vi "Translate 1D indexes to 2D.vi"(8 "error in (no error)":errorcluster, 10 "Range Array for Queue size mapping":refnum<class "2D Array s64.lvclass">, 11 "1D Indexes in":refnum<class "1D Array u32.lvclass">) -> (0 "error out":errorcluster, 3 "Mapped to 2D indexes out":refnum<class "1D Array s32.lvclass">)   [LabVIEW 2020, in "G2CPU Line Profile.lvlib"]
uses:
  G2CPU Line Profile.lvlib
  <vilib>/Natan Biesmans/G2CPU GPU and CPU HPC Toolkit/G2CPU Libraries/Arrays/1DArray/u32/1D Array u32.lvclass
  C:/Program Files/National Instruments/LabVIEW 2025/vi.lib/Natan Biesmans/G2CPU GPU and CPU HPC Toolkit/G2CPU Libraries/Arrays/Array/Array Prototype.lvclass
  <vilib>/Natan Biesmans/G2CPU GPU and CPU HPC Toolkit/G2CPU Libraries/Arrays/2DArray/s64/2D Array s64.lvclass
  <vilib>/Natan Biesmans/G2CPU GPU and CPU HPC Toolkit/G2CPU Libraries/Arrays/1DArray/s32/1D Array s32.lvclass
  <vilib>/Natan Biesmans/G2CPU GPU and CPU HPC Toolkit/G2CPU Libraries/Arrays/Array/Array Prototype.lvclass/Array Prototype.ctl
  3cda7c46-1737-42c5-90ff-c6c13540a65e.vi
  28bd746a-8bdf-434a-83c2-b49bf21645d8.vi
  78b6c921-1702-49f5-a8de-ca7d67101d2e.vi
  74281535-8ec9-475a-9c6f-61cdcc5771e7.vi
  da6a37ee-0c13-4542-a02e-82ed8c504917.vi
  f0154963-fb83-49e6-af23-53d56b8f6f43.vi
  fa8fd128-a982-493c-bb6b-fb6c2fa3ced3.vi
  dd97a9ad-5d19-4764-bb21-7805c3de5fd8.vi
  <vilib>/Natan Biesmans/G2CPU GPU and CPU HPC Toolkit/G2CPU Libraries/Arrays/Array/G2CPU Get Array Pointer.vi
  3cda7c46-1737-42c5-90ff-c6c13540a65e.vi/e7247370-a01f-465a-ac0e-4dfefcb1bb87.vi
  3cda7c46-1737-42c5-90ff-c6c13540a65e.vi/345e91f0-9a5e-4de4-af9c-133346717e4a.vi
  28bd746a-8bdf-434a-83c2-b49bf21645d8.vi/e7247370-a01f-465a-ac0e-4dfefcb1bb87.vi
  28bd746a-8bdf-434a-83c2-b49bf21645d8.vi/345e91f0-9a5e-4de4-af9c-133346717e4a.vi
  78b6c921-1702-49f5-a8de-ca7d67101d2e.vi/008596a2-72c7-4b94-8d63-a430db0cac39.vi
  78b6c921-1702-49f5-a8de-ca7d67101d2e.vi/d781c0aa-35dc-4978-ac14-8fc3832ba4f0.vi
  78b6c921-1702-49f5-a8de-ca7d67101d2e.vi/5ea8fe8e-4ffc-4d1c-84a0-6eba72fe9718.vi
  78b6c921-1702-49f5-a8de-ca7d67101d2e.vi/e2c9d363-485e-46f6-8192-2d8aa165dabd.vi
  78b6c921-1702-49f5-a8de-ca7d67101d2e.vi/677e326b-dc8f-4d68-b1d9-971c0162f72d.vi
  74281535-8ec9-475a-9c6f-61cdcc5771e7.vi/e2c9d363-485e-46f6-8192-2d8aa165dabd.vi
  74281535-8ec9-475a-9c6f-61cdcc5771e7.vi/677e326b-dc8f-4d68-b1d9-971c0162f72d.vi
  da6a37ee-0c13-4542-a02e-82ed8c504917.vi/5793b77b-c002-4ebf-9075-685617c95341.vi
  da6a37ee-0c13-4542-a02e-82ed8c504917.vi/2ed3ef86-c00d-4d71-b84c-20267a6dfcf9.vi
  f0154963-fb83-49e6-af23-53d56b8f6f43.vi/cfed8f62-9c64-4dab-912e-5e7c21cb720b.vi
  fa8fd128-a982-493c-bb6b-fb6c2fa3ced3.vi/5793b77b-c002-4ebf-9075-685617c95341.vi
  fa8fd128-a982-493c-bb6b-fb6c2fa3ced3.vi/2ed3ef86-c00d-4d71-b84c-20267a6dfcf9.vi
  dd97a9ad-5d19-4764-bb21-7805c3de5fd8.vi/9d769ba4-bbb4-4eb6-9175-95d7d139327c.vi
  dd97a9ad-5d19-4764-bb21-7805c3de5fd8.vi/8bfea9e7-a130-4d69-b32e-15c58d17157f.vi
  dd97a9ad-5d19-4764-bb21-7805c3de5fd8.vi/25f1b8bb-c437-45f4-b6eb-f3e32cc20aa5.vi
  dd97a9ad-5d19-4764-bb21-7805c3de5fd8.vi/309f54b5-9a40-4a1d-900d-2d620fefb202.vi
  da6a37ee-0c13-4542-a02e-82ed8c504917.vi/5793b77b-c002-4ebf-9075-685617c95341.vi/3e802c67-fb96-46a3-ae13-4994a8508b4f.vi
  da6a37ee-0c13-4542-a02e-82ed8c504917.vi/5793b77b-c002-4ebf-9075-685617c95341.vi/5a50fc67-79e7-4972-80c2-92243cd53dd4.vi
  da6a37ee-0c13-4542-a02e-82ed8c504917.vi/5793b77b-c002-4ebf-9075-685617c95341.vi/4b7910ad-0c4a-46e4-b1b3-c9721aeaa91e.vi
  da6a37ee-0c13-4542-a02e-82ed8c504917.vi/2ed3ef86-c00d-4d71-b84c-20267a6dfcf9.vi/730f6c57-5c0b-4ee9-b61e-75067b25222b.vi
  da6a37ee-0c13-4542-a02e-82ed8c504917.vi/2ed3ef86-c00d-4d71-b84c-20267a6dfcf9.vi/096b8799-7810-404e-baca-ba9279cec4bd.vi
  da6a37ee-0c13-4542-a02e-82ed8c504917.vi/2ed3ef86-c00d-4d71-b84c-20267a6dfcf9.vi/0f1a5a47-bcc5-4796-ac31-8dfcfbc0d7d1.vi
  da6a37ee-0c13-4542-a02e-82ed8c504917.vi/2ed3ef86-c00d-4d71-b84c-20267a6dfcf9.vi/89f12e17-3330-4b72-ad8f-8dd636660732.vi
  f0154963-fb83-49e6-af23-53d56b8f6f43.vi/cfed8f62-9c64-4dab-912e-5e7c21cb720b.vi/77c7badc-ed81-4514-99c1-20d37f4e5ecc.vi
  f0154963-fb83-49e6-af23-53d56b8f6f43.vi/cfed8f62-9c64-4dab-912e-5e7c21cb720b.vi/eb76fa01-6782-47b4-b34f-9eb474c9cc78.vi
  <vilib>/Natan Biesmans/G2CPU GPU and CPU HPC Toolkit/ArrayFire Driver/VIs/Run as Multi Device.vi
  fa8fd128-a982-493c-bb6b-fb6c2fa3ced3.vi/5793b77b-c002-4ebf-9075-685617c95341.vi/3e802c67-fb96-46a3-ae13-4994a8508b4f.vi
  fa8fd128-a982-493c-bb6b-fb6c2fa3ced3.vi/5793b77b-c002-4ebf-9075-685617c95341.vi/5a50fc67-79e7-4972-80c2-92243cd53dd4.vi
  fa8fd128-a982-493c-bb6b-fb6c2fa3ced3.vi/2ed3ef86-c00d-4d71-b84c-20267a6dfcf9.vi/730f6c57-5c0b-4ee9-b61e-75067b25222b.vi
  fa8fd128-a982-493c-bb6b-fb6c2fa3ced3.vi/2ed3ef86-c00d-4d71-b84c-20267a6dfcf9.vi/096b8799-7810-404e-baca-ba9279cec4bd.vi
  fa8fd128-a982-493c-bb6b-fb6c2fa3ced3.vi/2ed3ef86-c00d-4d71-b84c-20267a6dfcf9.vi/0f1a5a47-bcc5-4796-ac31-8dfcfbc0d7d1.vi
  fa8fd128-a982-493c-bb6b-fb6c2fa3ced3.vi/2ed3ef86-c00d-4d71-b84c-20267a6dfcf9.vi/89f12e17-3330-4b72-ad8f-8dd636660732.vi
  dd97a9ad-5d19-4764-bb21-7805c3de5fd8.vi/8bfea9e7-a130-4d69-b32e-15c58d17157f.vi/edd31282-7992-4bba-af75-482693dee5e1.vi
  dd97a9ad-5d19-4764-bb21-7805c3de5fd8.vi/309f54b5-9a40-4a1d-900d-2d620fefb202.vi/730f6c57-5c0b-4ee9-b61e-75067b25222b.vi
  dd97a9ad-5d19-4764-bb21-7805c3de5fd8.vi/309f54b5-9a40-4a1d-900d-2d620fefb202.vi/096b8799-7810-404e-baca-ba9279cec4bd.vi
  dd97a9ad-5d19-4764-bb21-7805c3de5fd8.vi/309f54b5-9a40-4a1d-900d-2d620fefb202.vi/0f1a5a47-bcc5-4796-ac31-8dfcfbc0d7d1.vi
  dd97a9ad-5d19-4764-bb21-7805c3de5fd8.vi/309f54b5-9a40-4a1d-900d-2d620fefb202.vi/89f12e17-3330-4b72-ad8f-8dd636660732.vi
  da6a37ee-0c13-4542-a02e-82ed8c504917.vi/5793b77b-c002-4ebf-9075-685617c95341.vi/5a50fc67-79e7-4972-80c2-92243cd53dd4.vi/1b7cf390-2ae0-48f3-9bce-03c57eed6ee8.vi
  <vilib>/Natan Biesmans/G2CPU GPU and CPU HPC Toolkit/G2CPU Libraries/Arrays/2DArray/s32/2D Array s32.lvclass
  <vilib>/Natan Biesmans/G2CPU GPU and CPU HPC Toolkit/ArrayFire Driver/VIs/cast.vi
  <vilib>/Natan Biesmans/G2CPU GPU and CPU HPC Toolkit/G2CPU Libraries/Arrays/Array/G2CPU Set Array Pointer.vi
  <vilib>/Natan Biesmans/G2CPU GPU and CPU HPC Toolkit/ArrayFire Driver/VIs/imax.vi
  <vilib>/Natan Biesmans/G2CPU GPU and CPU HPC Toolkit/G2CPU Libraries/Arrays/SubVI/RemoveReducedDimensionForReorder.vi
  <vilib>/Natan Biesmans/G2CPU GPU and CPU HPC Toolkit/ArrayFire Driver/VIs/reorder.vi
  <vilib>/Natan Biesmans/G2CPU GPU and CPU HPC Toolkit/ArrayFire Driver/VIs/release array.vi
  <vilib>/Natan Biesmans/G2CPU GPU and CPU HPC Toolkit/ArrayFire Driver/subvi/Error Converter (ErrCode or Status).vi
  <vilib>/Natan Biesmans/G2CPU GPU and CPU HPC Toolkit/G2CPU Libraries/Arrays/SubVI/is 1D.vi
  <vilib>/Natan Biesmans/G2CPU GPU and CPU HPC Toolkit/ArrayFire Driver/VIs/add.vi
  <vilib>/Natan Biesmans/G2CPU GPU and CPU HPC Toolkit/ArrayFire Driver/VIs/iszero.vi
  <vilib>/Natan Biesmans/G2CPU GPU and CPU HPC Toolkit/ArrayFire Driver/VIs/sub.vi
  <vilib>/Natan Biesmans/G2CPU GPU and CPU HPC Toolkit/ArrayFire Driver/VIs/mod.vi
  <vilib>/Natan Biesmans/G2CPU GPU and CPU HPC Toolkit/G2CPU Libraries/Arrays/Array/Array Prototype.lvclass
  <vilib>/Natan Biesmans/G2CPU GPU and CPU HPC Toolkit/G2CPU Libraries/Arrays/1DArray/1D Array Prototype.lvclass
  <vilib>/Natan Biesmans/G2CPU GPU and CPU HPC Toolkit/G2CPU Libraries/Arrays/2DArray/2D Array Prototype.lvclass
  <vilib>/Natan Biesmans/G2CPU GPU and CPU HPC Toolkit/G2CPU Libraries/Arrays/DataTypes/I32/s32.lvclass
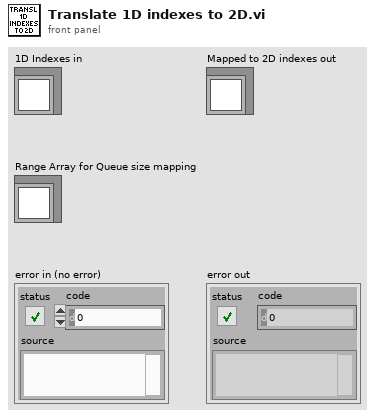
[diagram p1: front panel]
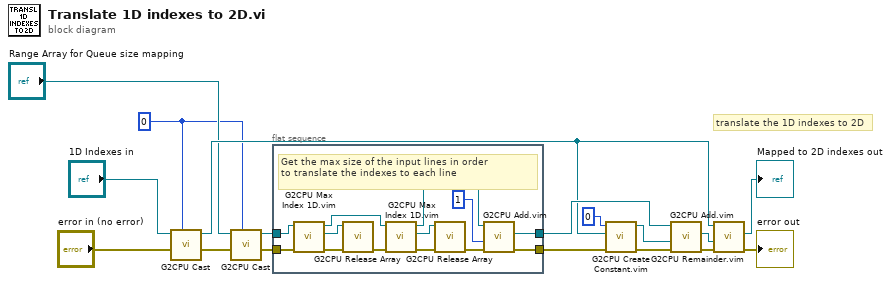
[diagram p0: block diagram]
diagram:
  w8 = 0 ("Datatype Prototype")
  # "translate the 1D indexes to 2D"
  n1 = call "G2CPU Cast"("Datatype Prototype"=w8, "error in (no error)"="error in (no error)", "Array In"="1D Indexes in") -> ("error out"=w10:errorcluster, "Array Out"=w11:refnum<class "1D Array s32.lvclass">)  [unwired: 7 in]
  n2 = call "G2CPU Cast"("Datatype Prototype"=w8, "error in (no error)"=w10, "Array In"="Range Array for Queue size mapping") -> ("error out"=w6:errorcluster, "Array Out"=w7:refnum<class "2D Array s32.lvclass">)  [unwired: 7 in]
  n3 = flat-sequence {
    tunnel: w6 -> [w24]
    tunnel: w7 -> [w23]
    tunnel: [w22] -> w12
    tunnel: [w21] -> w15
    frame #0 {
      # "Get the max size of the input lines in order\nto translate the indexes to each line"
      n4 = call "G2CPU Max Index 1D.vim"("error in (no error)"=w24, "Array First"=w23) -> ("error out"=w19:errorcluster, "Array idx"=w18:refnum<class "1D Array u32.lvclass">, "Array out"=w25:refnum<class "1D Array s32.lvclass">)  [unwired: 7 in]
      n5 = call <vilib>:"G2CPU Release Array.vi"("error in (no error)"=w19, "Array in"=w18) -> ("error out"=w27:errorcluster)  [unwired: 9 in]
      n6 = call "G2CPU Max Index 1D.vim"("error in (no error)"=w27, "Array First"=w25) -> ("error out"=w28:errorcluster, "Array idx"=w29:refnum<class "1D Array u32.lvclass">, "Array out"=w26:refnum<class "1D Array s32.lvclass">)  [unwired: 7 in]
      n7 = call <vilib>:"G2CPU Release Array.vi"("error in (no error)"=w28, "Array in"=w29) -> ("error out"=w30:errorcluster)  [unwired: 9 in]
      n8 = call "G2CPU Add.vim"("error in (no error)"=w30, "Array rhs"=1 ("Datatype Prototype"), "Array lhs"=w26) -> ("error out"=w21:errorcluster, "Array Result"=w22:refnum<class "1D Array s32.lvclass">)  [unwired: 7 in]
    }
  }
  n9 = call "G2CPU Create Constant.vim"("error in (no error)"=w15, "Size"=w11, "val"=0) -> ("error out"=w14:errorcluster, "object out"=w13:refnum<class "1D Array s32.lvclass">)  [unwired: 7 in]
  n10 = call "G2CPU Add.vim"("error in (no error)"=w14, "Array rhs"=w13, "Array lhs"=w12) -> ("error out"=w2:errorcluster, "Array Result"=w1:refnum<class "1D Array s32.lvclass">)  [unwired: 7 in]
  n11 = call "G2CPU Remainder.vim"("error in (no error)"=w2, "Array rhs"=w1, "Array lhs"=w11) -> ("error out"=→"error out":errorcluster, "Array Result"=→"Mapped to 2D indexes out":refnum<class "1D Array s32.lvclass">)  [unwired: 7 in]
